vi "testParseStateQueueInlining.vi"(8 "error in (no error)":errorcluster, 11 "testStateMachineUtilities in":refnum<class "testStateMachineUtilities.lvclass">=refnum) -> (0 "error out":errorcluster, 3 "testStateMachineUtilities out":refnum<class "testStateMachineUtilities.lvclass">)   [LabVIEW 2016, in "testStateMachineUtilities.lvclass"]
uses:
  testStateMachineUtilities.lvclass
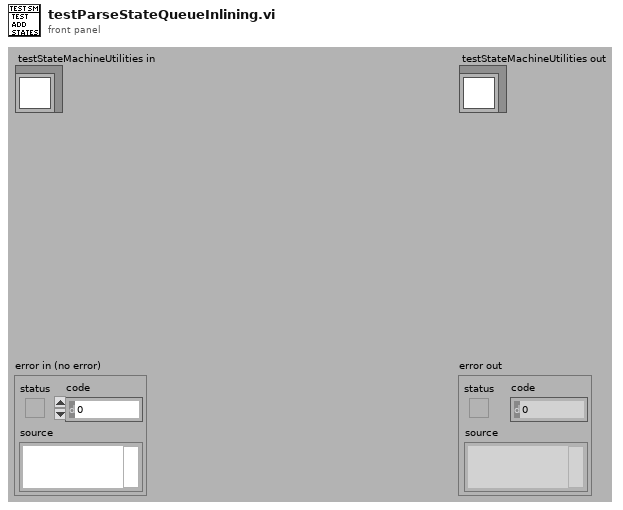
[diagram p1: front panel]
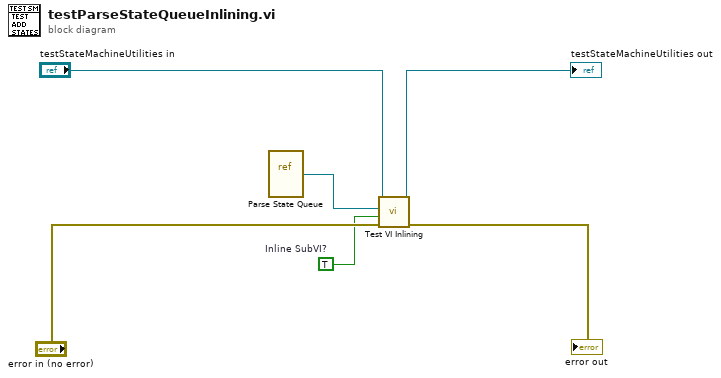
[diagram p0: block diagram]
diagram:
  w1 = TRUE  # Inline SubVI?
  n1 = vi-ref "Parse State Queue.vi"() -> (w6:refnum<vi>)
  n2 = call "Test VI Inlining.vi"("error in (no error)"="error in (no error)", "Inline SubVI?"=w1, "VI Refnum"=w6, "testStateMachineUtilities in"="testStateMachineUtilities in") -> ("error out"=→"error out":errorcluster, "testStateMachineUtilities out"=→"testStateMachineUtilities out":refnum<class "testStateMachineUtilities.lvclass">)  [unwired: 6 in]
